vi "FormIO.vi"() -> ()   [LabVIEW 2013]
uses:
  S7Ref.vi
panel:
  out "DI 4":T1
  out "DI 5":T1
  in  "DQ 4":T1
  in  "DQ 5":T1
  in  "DQ 6":T2
  in  "选项卡控件":enum32{"开关信号/操作", "传感器信号"}(tab)
  out "DI 0":T3
  out "DI 2":T4
  out "DI 1":T5
  out "DI 3":T6
  in  "DQ 0":T7
  in  "DQ 1":T1
  in  "DQ 2":T8
  in  "DQ 3":T1
  out "AI":T9 {"V    AI 7" format="%#.2g"; "V    AI 6" format="%#.2g"; "V    AI 5" format="%#.2g"; "V    AI 4" format="%#.2g"; "V    AI 3" format="%#.2g"; "V    AI 2" format="%#.2g"; "V    AI 1" format="%#.2g"; "V    AI 0" format="%#.2g"}
  # "输入上"
  # "输入下"
  # "输出上"
  # "输出下"
  # "输入正"
  # "输入反"
  # "输出正"
  # "输出反"
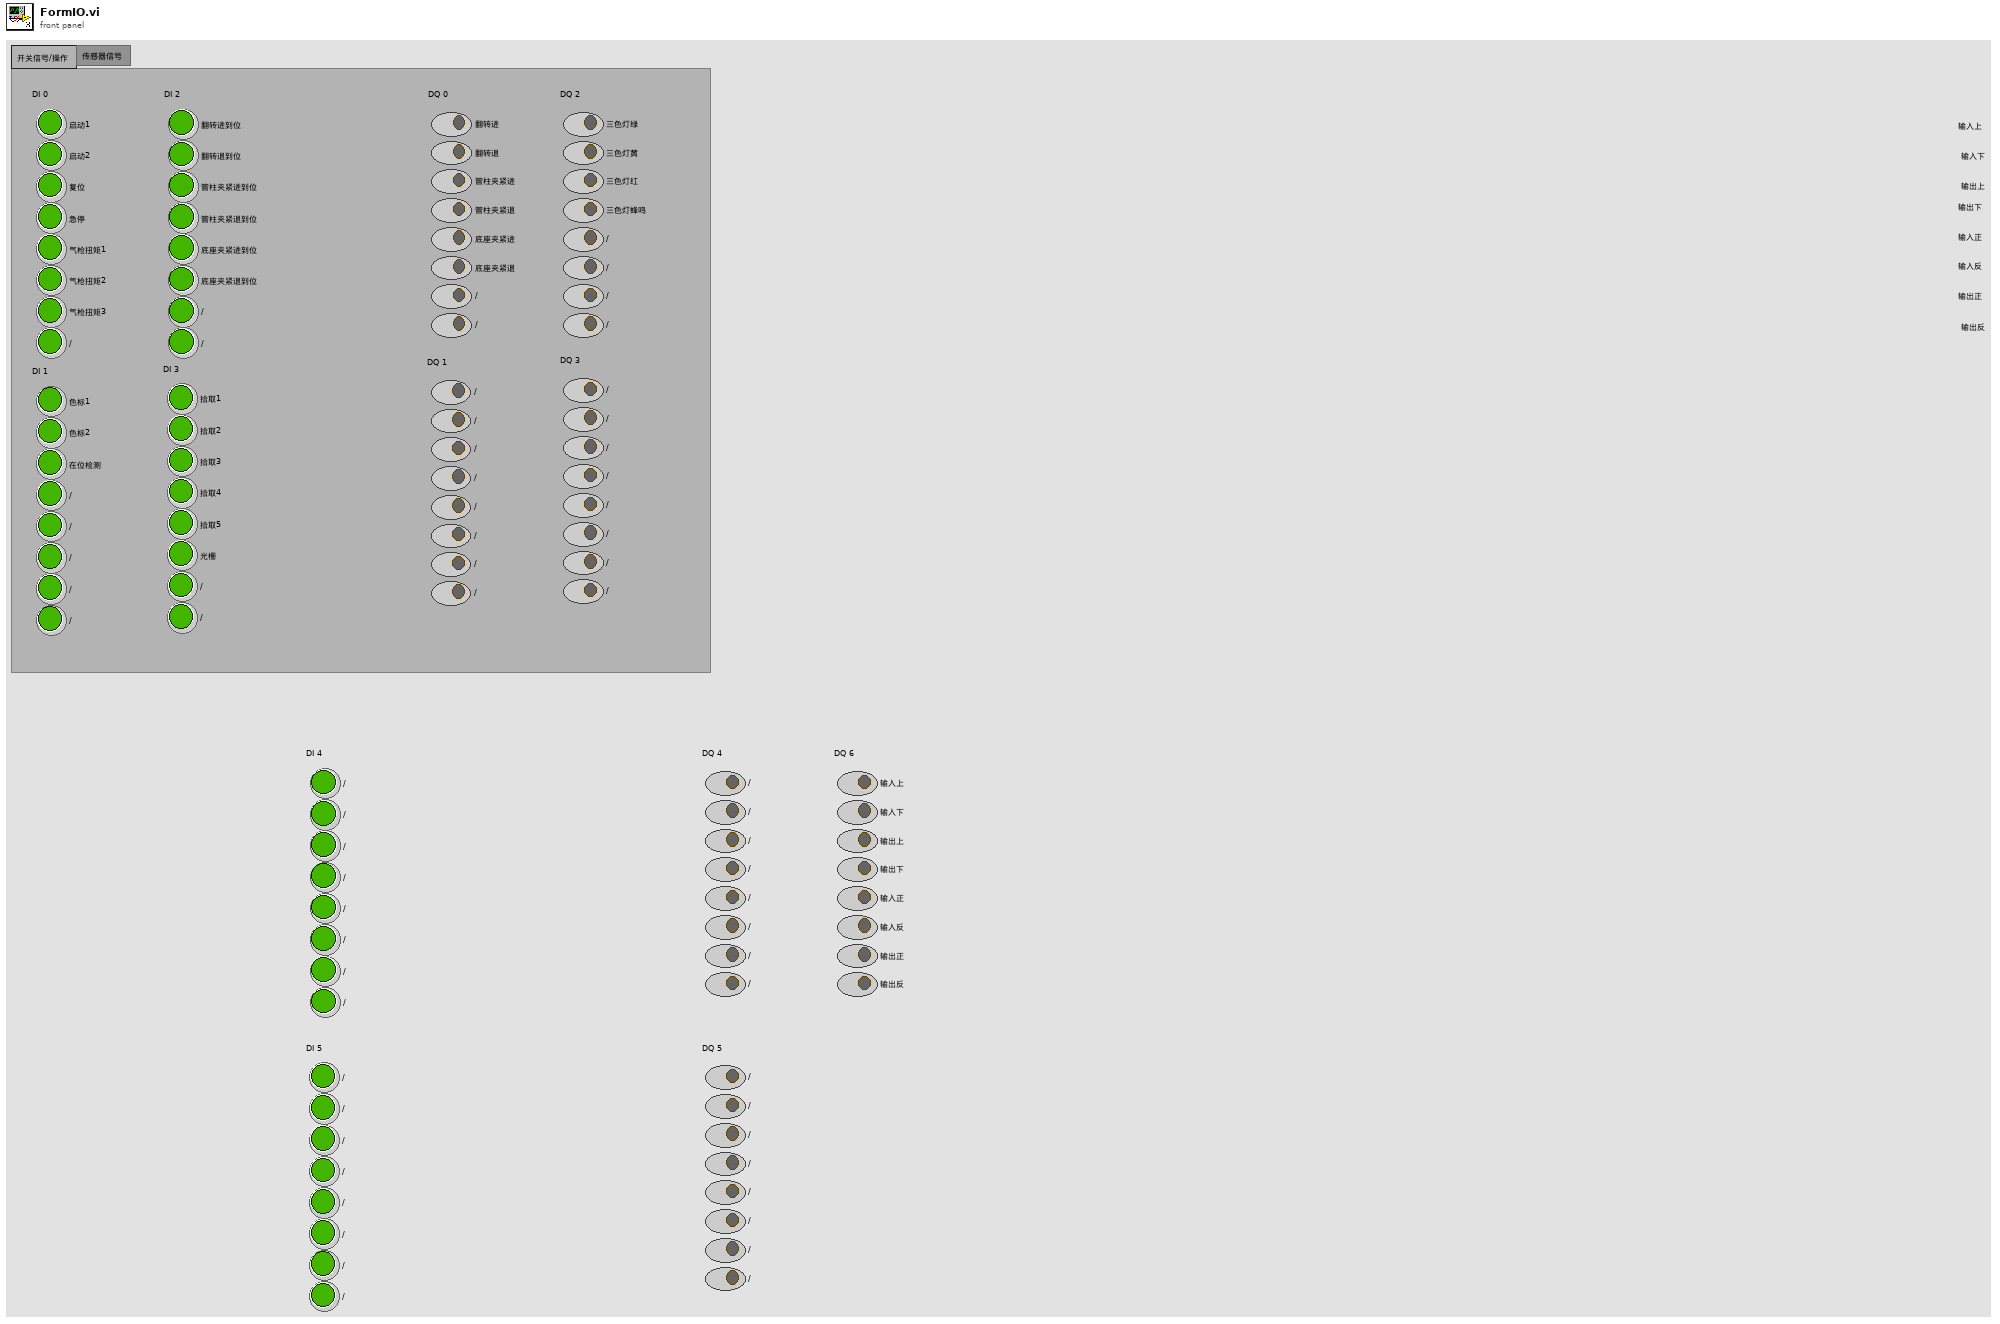
[diagram p1: front panel]
types:
  T1 = cluster{"/":bool, "/":bool, "/":bool, "/":bool, "/":bool, "/":bool, "/":bool, "/":bool}
  T2 = cluster{"输入上":bool, "输入下":bool, "输出上":bool, "输出下":bool, "输入正":bool, "输入反":bool, "输出正":bool, "输出反":bool}
  T3 = cluster{"启动1":bool, "启动2":bool, "复位":bool, "急停":bool, "气枪扭矩1":bool, "气枪扭矩2":bool, "气枪扭矩3":bool, "/":bool}
  T4 = cluster{"翻转进到位":bool, "翻转退到位":bool, "管柱夹紧进到位":bool, "管柱夹紧退到位":bool, "底座夹紧进到位":bool, "底座夹紧退到位":bool, "/":bool, "/":bool}
  T5 = cluster{"色标1":bool, "色标2":bool, "在位检测":bool, "/":bool, "/":bool, "/":bool, "/":bool, "/":bool}
  T6 = cluster{"拾取1":bool, "拾取2":bool, "拾取3":bool, "拾取4":bool, "拾取5":bool, "光栅":bool, "/":bool, "/":bool}
  T7 = cluster{"翻转进":bool, "翻转退":bool, "管柱夹紧进":bool, "管柱夹紧退":bool, "底座夹紧进":bool, "底座夹紧退":bool, "/":bool, "/":bool}
  T8 = cluster{"三色灯绿":bool, "三色灯黄":bool, "三色灯红":bool, "三色灯蜂鸣":bool, "/":bool, "/":bool, "/":bool, "/":bool}
  T9 = cluster{"V    AI 0":dbl, "V    AI 1":dbl, "V    AI 2":dbl, "V    AI 3":dbl, "V    AI 4":dbl, "V    AI 5":dbl, "V    AI 6":dbl, "V    AI 7":dbl}
  T10 = cluster{"输入移正脉冲":bool, "输入移反脉冲":bool, "输出移正脉冲":bool, "输出移反脉冲":bool, "控制器转速":bool, "/":bool, "控制器车速":bool, "/":bool}
  T11 = cluster{bool, bool, bool, bool, bool, bool, bool, bool}
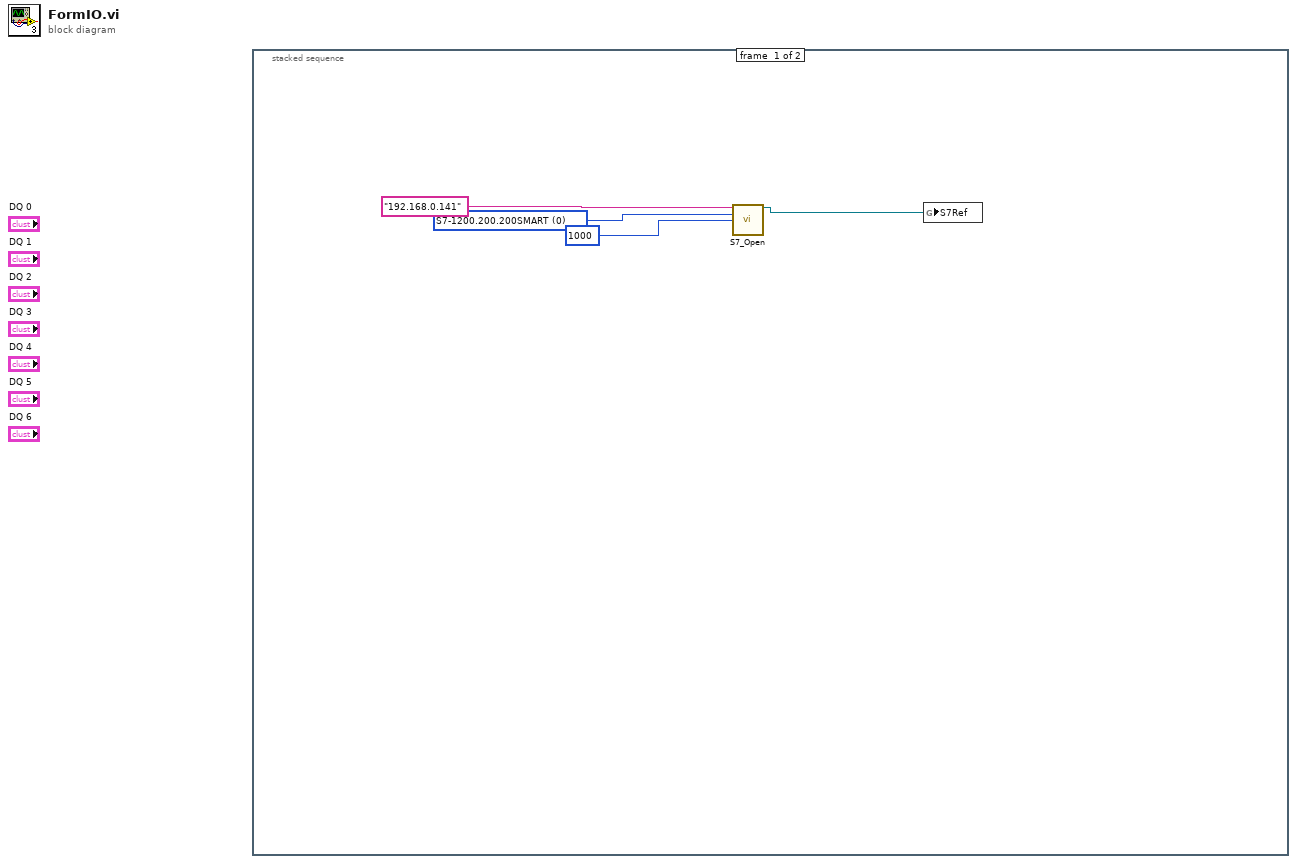
[diagram p0: block diagram]
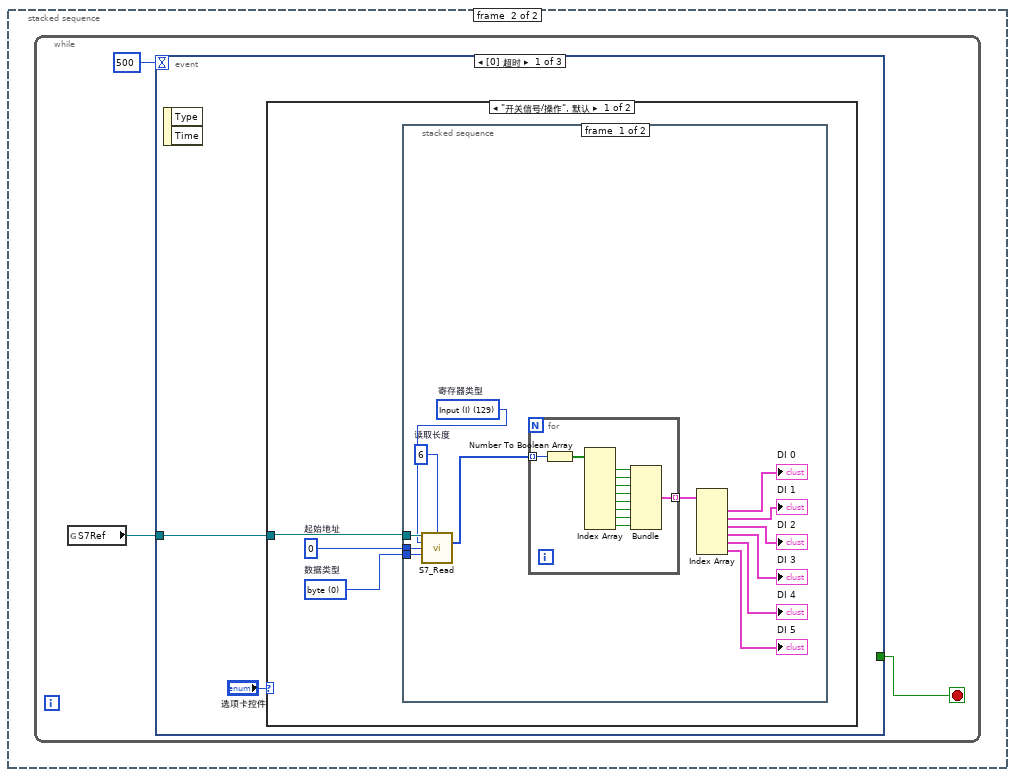
[diagram p2: hidden frame]
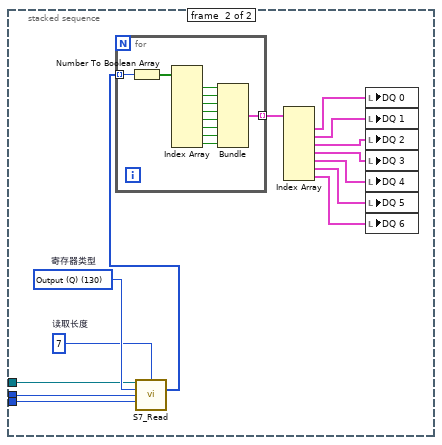
[diagram p3: hidden frame]
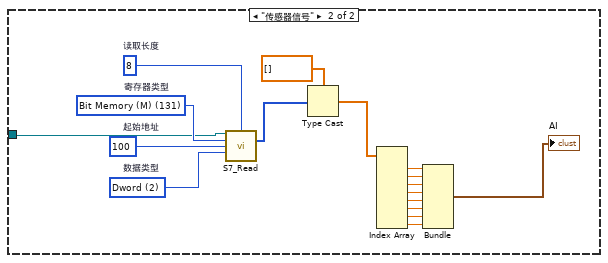
[diagram p4: hidden frame]
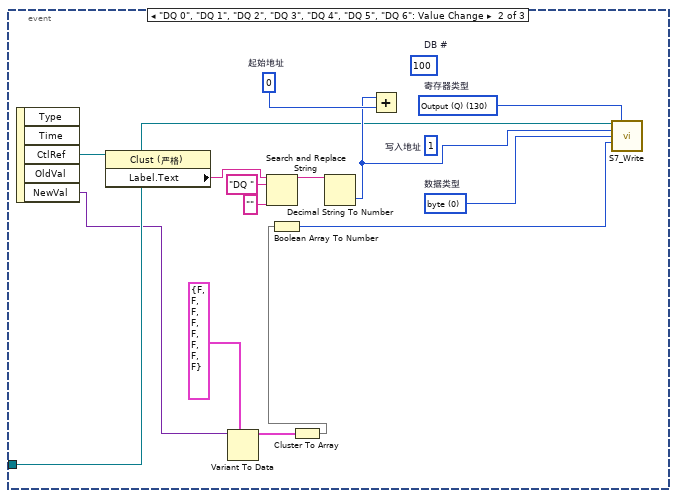
[diagram p5: hidden frame]
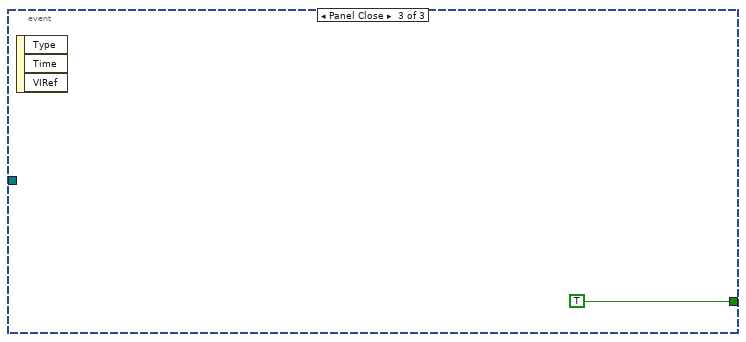
[diagram p6: hidden frame]
diagram:
  n1 = stacked-sequence {
    frame #0 {
      w3 = u8 0 items=["S7-1200.200.200SMART"=0, "S7-300"=2, "S7-400"=3] ("PLC 系列")
      n2 = call "S7_Open .vi"("IP 地址"="192.168.0.141", "PLC 系列"=w3, "超时（MS）"=1000) -> ("TCP"=w1:refnum<k5>)  [unwired: 9 in, 3 out]
      n3 = global write "S7Ref.vi" "S7Ref"(w1) -> ()
    }
    frame #1 {
      n4 = while {
        stop <- w7 stop-if-true
        n5 = global read "S7Ref.vi" "S7Ref"() -> (w5:refnum<k5>)
        n6 = event shown="[0] 超时" {
          selector: _ -> [_ _ _]
          dyn-events: _ -> [_ _ _]
          timeout: 500 -> [_ _ _]
          tunnel: [_ _ TRUE ("布尔")] -> w7
          tunnel: w5 -> [w8 w87 _]
          event Timeout {
            n7 = event-data() -> ()  [unwired: 1 in, 2 out]
            n8 = case shown="\"开关信号/操作\", 默认" "选项卡控件" {
              tunnel: w8 -> [w12 w73]
              frame "开关信号/操作", Default {
                w10 = u16 0 items=["byte", "word", "Dword"]  # 数据类型
                w11 = u32 0  # 起始地址
                n9 = stacked-sequence {
                  tunnel: w12 -> [w25 w49]
                  tunnel: w11 -> [w24 w48]
                  tunnel: w10 -> [w23 w47]
                  frame #0 {
                    w13 = u16 6  # 读取长度
                    w22 = u8 129 items=["I/O (P)"=128, "Input (I)"=129, "Output (Q)"=130, "Bit Memory (M)"=131, "Data (DB)"=132, "Instance Data (DI)"=133, "Local Data (L)"=134, "Predecessor Local Data (VL)"=135]  # 寄存器类型
                    n10 = call "S7_Read .vi"("TCP"=w25, "读取长度"=w13, "寄存器类型"=w22, "起始地址"=w24, "数据类型"=w23) -> ("数据"=w21:u32[])  [unwired: 7 in, 3 out]
                    n11 = for {
                      tunnel: w21 -> [w36] mode=indexing
                      tunnel: [w26] -> w20 mode=indexing
                      n12 = Number To Boolean Array(number=w36) -> (Boolean array=w35:bool[])
                      n13 = Index Array(array=w35) -> (element #1=w34:bool, element #2=w33:bool, element #3=w32:bool, element #4=w31:bool, element #5=w30:bool, element #6=w29:bool, element #7=w28:bool, element #8=w27:bool)  [unwired: 8 in]
                      n14 = Bundle(w34, w33, w32, w31, w30, w29, w28, w27) -> (w26:T11)  [unwired: 1 in]
                    }
                    n15 = Index Array(array=w20) -> (element #1=→"DI 0":T11, element #2=→"DI 1":T11, element #3=→"DI 2":T11, element #4=→"DI 3":T11, element #5=→"DI 4":T11, element #6=→"DI 5":T11)  [unwired: 6 in]
                  }
                  frame #1 {
                    w37 = u16 7  # 读取长度
                    w50 = u8 130 items=["I/O (P)"=128, "Input (I)"=129, "Output (Q)"=130, "Bit Memory (M)"=131, "Data (DB)"=132, "Instance Data (DI)"=133, "Local Data (L)"=134, "Predecessor Local Data (VL)"=135]  # 寄存器类型
                    n16 = call "S7_Read .vi"("TCP"=w49, "读取长度"=w37, "寄存器类型"=w50, "起始地址"=w48, "数据类型"=w47) -> ("数据"=w45:u32[])  [unwired: 7 in, 3 out]
                    n17 = for {
                      tunnel: w45 -> [w61] mode=indexing
                      tunnel: [w51] -> w46 mode=indexing
                      n18 = Number To Boolean Array(number=w61) -> (Boolean array=w60:bool[])
                      n19 = Index Array(array=w60) -> (element #1=w59:bool, element #2=w58:bool, element #3=w57:bool, element #4=w56:bool, element #5=w55:bool, element #6=w54:bool, element #7=w53:bool, element #8=w52:bool)  [unwired: 8 in]
                      n20 = Bundle(w59, w58, w57, w56, w55, w54, w53, w52) -> (w51:T11)  [unwired: 1 in]
                    }
                    n21 = Index Array(array=w46) -> (element #1=w44:T11, element #2=w43:T11, element #3=w42:T11, element #4=w41:T11, element #5=w40:T11, element #6=w39:T11, element #7=w38:T11)  [unwired: 7 in]
                    n22 = local write "DQ 0"(w44) -> ()
                    n23 = local write "DQ 1"(w43) -> ()
                    n24 = local write "DQ 2"(w42) -> ()
                    n25 = local write "DQ 3"(w41) -> ()
                    n26 = local write "DQ 4"(w40) -> ()
                    n27 = local write "DQ 5"(w39) -> ()
                    n28 = local write "DQ 6"(w38) -> ()
                  }
                }
              }
              frame "传感器信号" {
                w76 = u16 2 items=["byte", "word", "Dword"]  # 数据类型
                w77 = u32 100  # 起始地址
                w78 = u8 131 items=["I/O (P)"=128, "Input (I)"=129, "Output (Q)"=130, "Bit Memory (M)"=131, "Data (DB)"=132, "Instance Data (DI)"=133, "Local Data (L)"=134, "Predecessor Local Data (VL)"=135]  # 寄存器类型
                w75 = u16 8  # 读取长度
                n29 = call "S7_Read .vi"("TCP"=w73, "读取长度"=w75, "寄存器类型"=w78, "起始地址"=w77, "数据类型"=w76) -> ("数据"=w72:u32[])  [unwired: 7 in, 3 out]
                n30 = Type Cast(type=sgl[] [] ("添加的数组"), x=w72) -> (*(type *) &x=w63:sgl[])
                n31 = Index Array(array=w63) -> (element #1=w64:sgl, element #2=w65:sgl, element #3=w66:sgl, element #4=w67:sgl, element #5=w68:sgl, element #6=w69:sgl, element #7=w70:sgl, element #8=w71:sgl)  [unwired: 8 in]
                n32 = Bundle(w64, w65, w66, w67, w68, w69, w70, w71) -> (→"AI":cluster{sgl, sgl, sgl, sgl, sgl, sgl, sgl, sgl})  [unwired: 1 in]
              }
            }
          }
          event "DQ 0", "DQ 1", "DQ 2", "DQ 3", "DQ 4", "DQ 5", "DQ 6": Value Change {
            w90 = u32 0  # 起始地址
            w92 = u16 0 items=["byte", "word", "Dword"]  # 数据类型
            (unwired) u32 1  # 写入地址
            (unwired) u16 100  # DB #
            w93 = u8 130 items=["I/O (P)"=128, "Input (I)"=129, "Output (Q)"=130, "Bit Memory (M)"=131, "Data (DB)"=132, "Instance Data (DI)"=133, "Local Data (L)"=134, "Predecessor Local Data (VL)"=135]  # 寄存器类型
            n33 = event-data() -> ("CtlRef"=w89:refnum<vi>, "NewVal"=w85:variant)  [unwired: 1 in, 3 out]
            n34 = property class="Clust (严格)"(reference=w89) -> ("Label.Text"=w80:string)  [unwired: 1 in, 2 out]
            n35 = Variant To Data(type=T10 {"输入移正脉冲"=FALSE, "输入移反脉冲"=FALSE, "输出移正脉冲"=FALSE, "输出移反脉冲"=FALSE, "控制器转速"=FALSE, "/"=FALSE, "控制器车速"=FALSE, "/"=FALSE} ("DQ 0"), Variant=w85) -> (data=w84:T10)  [unwired: 1 in, 1 out]
            n36 = Search and Replace String(input string=w80, search string="DQ " ("搜索字符串"), replace string="" ("替换字符串(\"\")")) -> (result string=w79:string)  [unwired: 5 in, 3 out]
            n37 = Cluster To Array(cluster=w84) -> (array=w83:bool[])
            n38 = Boolean Array To Number ("布尔数组至数值转换")(Boolean array=w83) -> (number=w91:u8)
            n39 = Decimal String To Number(string=w79) -> (number=w88:i32)  [unwired: 2 in, 1 out]
            n40 = Add(x=w88, y=w90) -> ()  [unwired: 1 out]
            n41 = call "S7_Write .vi"("TCP"=w87, "寄存器类型"=w93, "写入地址"=w88, "数据类型"=w92, "写入数据"=w91) -> ()  [unwired: 8 in, 3 out]
          }
          event Panel Close {
            n42 = event-data() -> ()  [unwired: 1 in, 3 out]
          }
        }
      }
    }
  }
